vi "SVT Peak Level (1 Ch).vi"(6 "restart averaging (F)":bool, 8 "error in (no error)":errorcluster, 11 "scaled signal [EU]":waveform(dbl)) -> (0 "error out":errorcluster, 2 "unit label":string, 3 "peak level [EU]":dbl=nan format="%.2f")   [LabVIEW 2017]
doc: "Computes the peak level of <B>scaled signal [EU]</B> or <B>even angle signal [EU]</B>. You can use this polymorphic VI to compute the peak level for a single channel or for N channels, or for a single channel or N channels of angular resampled data. The data type you wire to the <B>scaled signal [EU]</B> or <B>even angle signal [EU]</B> input determines the polymorphic instance to use."
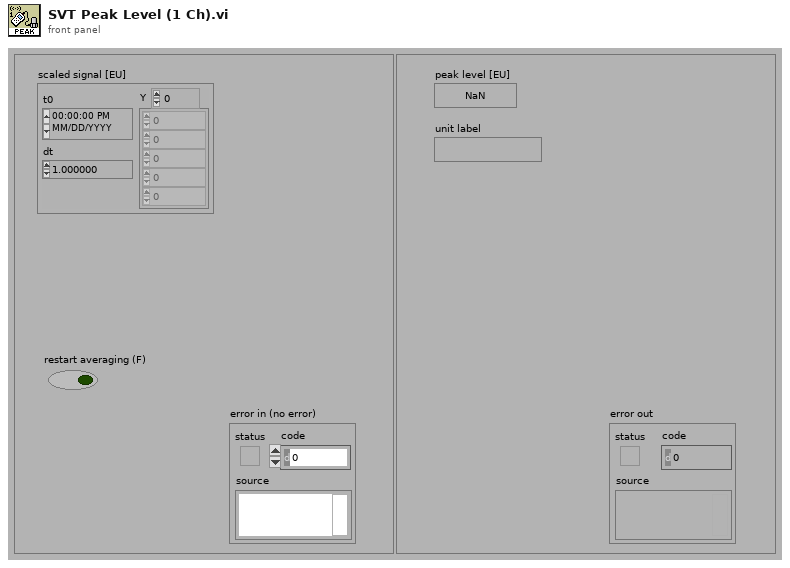
[diagram p1: front panel]
types:
  T1 = enum16{"RMS", "Running RMS", "Exp avg  ", "Dec exp avg ", "Peak", "Crest"}
  T2 = enum16{"Reset filter", "Restart averaging", "Continue processing"}
  T3 = typedef "svc_Channel Info.ctl" = cluster{"sensor sensitivity":dbl, "engineering units":T4, "dB reference":dbl, "custom label":string, "weighting filter":T5, "pregain":dbl}
  T4 = typedef "svc_Engineering Units Text Ring.ctl" = u16
  T5 = typedef "svc_Weighting Filter Text Ring.ctl" = u16
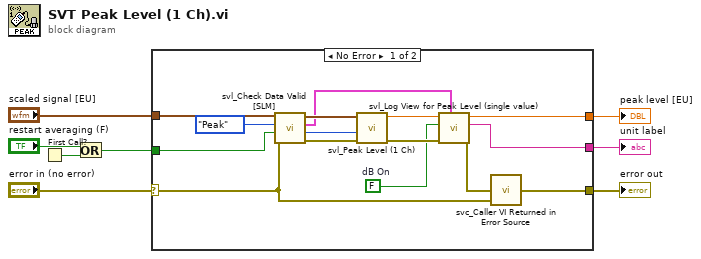
[diagram p0: block diagram]
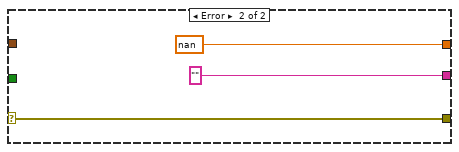
[diagram p2: hidden frame]
diagram:
  n1 = First Call?() -> (First Call?: T/F=w3:bool)
  n2 = Or(x="restart averaging (F)", y=w3) -> (x .or. y?=w1:bool)
  n3 = case shown="No Error" "error in (no error)" {
    tunnel: [w21 nan ("energy level [EU^2 rms]")] -> w6
    tunnel: [w20 "" ("unit label")] -> w5
    tunnel: "scaled signal [EU]" -> [w12 _]
    tunnel: w1 -> [w15 _]
    selector: "error in (no error)" -> [w9 w26]
    tunnel: [w22 w26] -> w8
    frame No Error {
      w13 = FALSE  # dB On
      n4 = call <vilib>:"svl_Check Data Valid [SLM].vi"("error in (no error)"=w9, "restart averaging (F)"=w15, "Level Analysis"=T1."Peak", "scaled signal [EU]"=w12) -> ("error out"=w17:errorcluster, "processing state"=w16:T2, "channel info"=w10:T3, "dup scaled signal [EU]"=w11:waveform(dbl))  [unwired: 4 in]
      n5 = call <vilib>:"svl_Peak Level (1 Ch).vi"("error in (no error)"=w17, "processing state"=w16, "scaled signal"=w11) -> ("error out"=w19:errorcluster, "peak level"=w18:dbl)  [unwired: 7 in]
      n6 = call <vilib>:"svl_Log View for Peak Level (single value).vi"("channel info"=w10, "error in (no error)"=w19, "dB On (T)"=w13, "peak level [EU]"=w18) -> ("error out"=w23:errorcluster, "unit label"=w20:string, "peak level [EU]"=w21:dbl)  [unwired: 5 in]
      n7 = call <vilib>:"svc_Caller VI Returned in Error Source.vi"("warning input to caller"=w9, "error in (no error)"=w23) -> ("error out"=w22:errorcluster)  [unwired: 3 in]
    }
    frame Error {
    }
  }
  "peak level [EU]" <- w6
  "unit label" <- w5
  "error out" <- w8
